vi "GetMetronome.vi"(11 "SendMsg.lvlib:Send.lvclass":refnum<class "Send.lvclass">) -> (3 "Metronome.lvclass":refnum<class "Metronome.lvclass">)   [LabVIEW 2019, in "UseMetronome.lvlib"]
uses:
  UseMetronome.lvlib
  Metronome.lvclass
  Send.lvclass
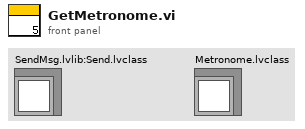
[diagram p1: front panel]
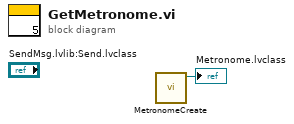
[diagram p0: block diagram]
diagram:
  n1 = call "MetronomeCreate.vi"() -> ("Metronome.lvclass"=→"Metronome.lvclass":refnum<class "Metronome.lvclass">)  [unwired: 11 in]
